vi "Tribot Dashboard.vi"() -> ()   [LabVIEW 2015, in "ExemploFinal.lvrbt"]
doc: "This VI allows you to drive all motors and view all sensor data for the NXT/EV3 Tribot configuration. This VI is designed to run targeted to the computer so you can view all your sensor data. You can build your own dashboad if you change the configuration."
uses:
  ExemploFinal.lvrbt
  <vilib>/NXT/Subs/MotorOutput.ctl
  <vilib>/NXT/Block Support/NXT_InputPort.ctl
  <vilib>/NXT/Dual Mode Library/Display/drawText.vi
  <vilib>/NXT/Dual Mode Library/Motors/MotorOn.vi
  <vilib>/NXT/Dual Mode Library/Sensors/Touch_Pressed.vi
  <vilib>/NXT/Dual Mode Library/Sensors/Sound_dB.vi
  <vilib>/NXT/Dual Mode Library/Sensors/Light_On.vi
  <vilib>/NXT/Dual Mode Library/Sensors/Sonar_cm.vi
  <vilib>/NXT/Dual Mode Library/Motors/MotorBrake.vi
panel:
  in  "?":string="Running LabVIEW  Dashboard\n\nPush orange\nbutton to stop"
  in  "Grabber":i32(slide) scale=-100.0..100.0
  out "Touch Sensor Pressed (Port 1)":bool
  out "Sound dB (Port 2)":i16(graph)
  out "Ultrasonic Sensor Data (Port 4)":i16(graph)
  out "Light Sensor Data (Port 3)":i16(graph)
  in  "Left Wheel":i32(slide) scale=-100.0..100.0
  in  "Right Wheel":i32(slide) scale=-100.0..100.0
  in  "Stop":bool
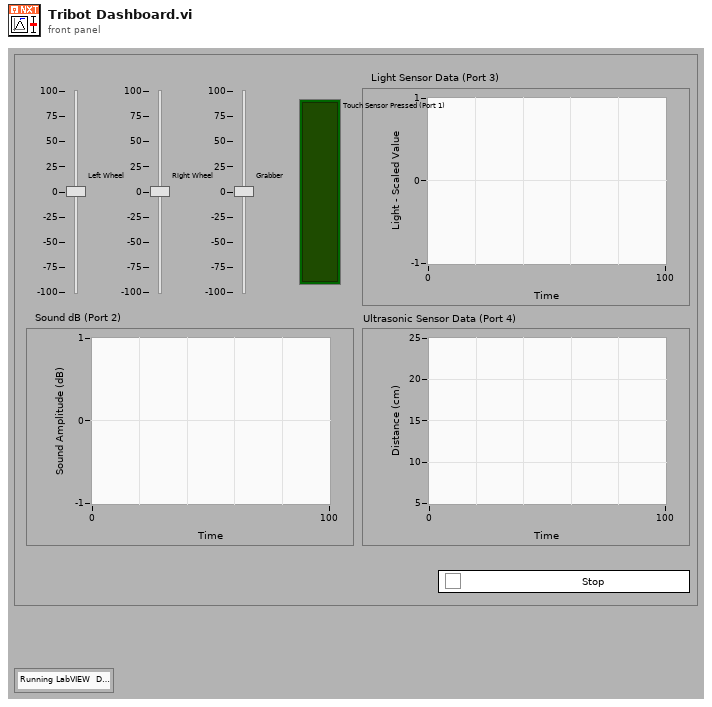
[diagram p1: front panel]
types:
  T1 = typedef "LVHSConnector.ctl" = refnum<class "BrickReference.lvclass">
  T2 = typedef "NXT_InputPort.ctl" = u32
  T3 = typedef "MotorOutput.ctl" = u8
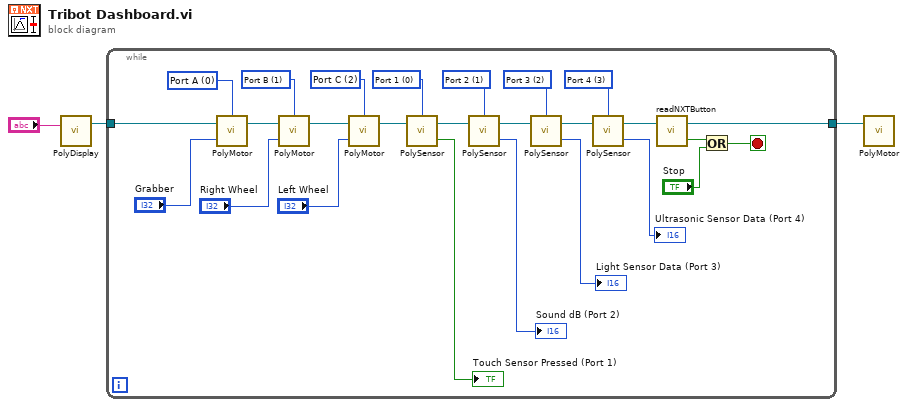
[diagram p0: block diagram]
diagram:
  n1 = call-poly <vilib>:"PolyDisplay.vi"("Text"="?") -> ("NXT/EV3"=w2:T1)  [unwired: 3 in]
  n2 = while {
    tunnel: w2 -> [w12]
    tunnel: [w4] -> w1
    stop <- w15 stop-if-true
    w28 = T2 2 items=["Port 1", "Port 2", "Port 3", "Port 4"] ("Port (Port 3)")
    w26 = T2 1 items=["Port 1", "Port 2", "Port 3", "Port 4"] ("Port (Port 2)")
    w24 = T2 3 items=["Port 1", "Port 2", "Port 3", "Port 4"] ("Port (Port 4)")
    w23 = T2 0 items=["Port 1", "Port 2", "Port 3", "Port 4"] ("Port (Port 1)")
    w21 = T3 0 items=["Port A"=0, "Port B"=1, "Port C"=2, "Ports A & B"=4, "Ports A & C"=5, "Ports B & C"=6, "All Ports"=3] ("Output Port (All Ports)")
    w18 = T3 1 items=["Port A"=0, "Port B"=1, "Port C"=2, "Ports A & B"=4, "Ports A & C"=5, "Ports B & C"=6, "All Ports"=3] ("Output Port (All Ports)")
    w17 = T3 2 items=["Port A"=0, "Port B"=1, "Port C"=2, "Ports A & B"=4, "Ports A & C"=5, "Ports B & C"=6, "All Ports"=3] ("Output Port (All Ports)")
    n3 = call-poly <vilib>:"PolyMotor.vi"("Power (75)"="Grabber", "NXT/EV3"=w12, "Output Port (All Ports)"=w21) -> ("NXT/EV3"=w11:T1)  [unwired: 1 in]
    n4 = call-poly <vilib>:"PolyMotor.vi"("Power (75)"="Right Wheel", "NXT/EV3"=w11, "Output Port (All Ports)"=w18) -> ("NXT/EV3"=w10:T1)  [unwired: 1 in]
    n5 = call-poly <vilib>:"PolyMotor.vi"("Power (75)"="Left Wheel", "NXT/EV3"=w10, "Output Port (All Ports)"=w17) -> ("NXT/EV3"=w9:T1)  [unwired: 1 in]
    n6 = call-poly <vilib>:"PolySensor.vi"("NXT/EV3"=w9, "Port (Port 1)"=w23) -> ("Yes / No"=→"Touch Sensor Pressed (Port 1)":bool, "NXT/EV3"=w8:T1)  [unwired: 1 in]
    n7 = call-poly <vilib>:"PolySensor.vi"("NXT/EV3"=w8, "Port (Port 2)"=w26) -> ("Sound (dB)"=→"Sound dB (Port 2)":i16, "NXT/EV3"=w7:T1)  [unwired: 1 in]
    n8 = call-poly <vilib>:"PolySensor.vi"("NXT/EV3"=w7, "Port (Port 3)"=w28) -> ("Scaled Value"=→"Light Sensor Data (Port 3)":i16, "NXT/EV3"=w6:T1)  [unwired: 1 in]
    n9 = call-poly <vilib>:"PolySensor.vi"("NXT/EV3"=w6, "Port (Port 4)"=w24) -> ("Distance (cm)"=→"Ultrasonic Sensor Data (Port 4)":i16, "NXT/EV3"=w5:T1)  [unwired: 1 in]
    n10 = call <vilib>:"readNXTButton.vi"("NXT/EV3"=w5) -> ("Yes/No"=w14:bool, "NXT/EV3"=w4:T1)  [unwired: 2 in]
    n11 = Or(x=w14, y="Stop") -> (x .or. y?=w15:bool)
  }
  n12 = call-poly <vilib>:"PolyMotor.vi"("NXT/EV3"=w1) -> ()  [unwired: 3 in, 1 out]
